vi "Set Z-plane selector disabled state.vi"(8 "error in (no error)":errorcluster, 11 "Functional Imging UI Refs":T1) -> (0 "error out":errorcluster)   [LabVIEW 2013]
uses:
  Typedefs/Functional Imging UI Refs.ctl
  xcontrol/XGrapher.xctl
  Typedefs/ROI selector array-ROI vis.ctl
  xcontrol/Interface VIs/Interface typedefs/Interface-ROI selection cluster.ctl
  Typedefs/ROI ID Enum.ctl
  Typedefs/Groups array referecne.ctl
  Typedefs/ROI visibility mode.ctl
  Global variables/gl_Functional Imaging-Global variables.vi
panel:
  # "[Groups] is a Typedef"
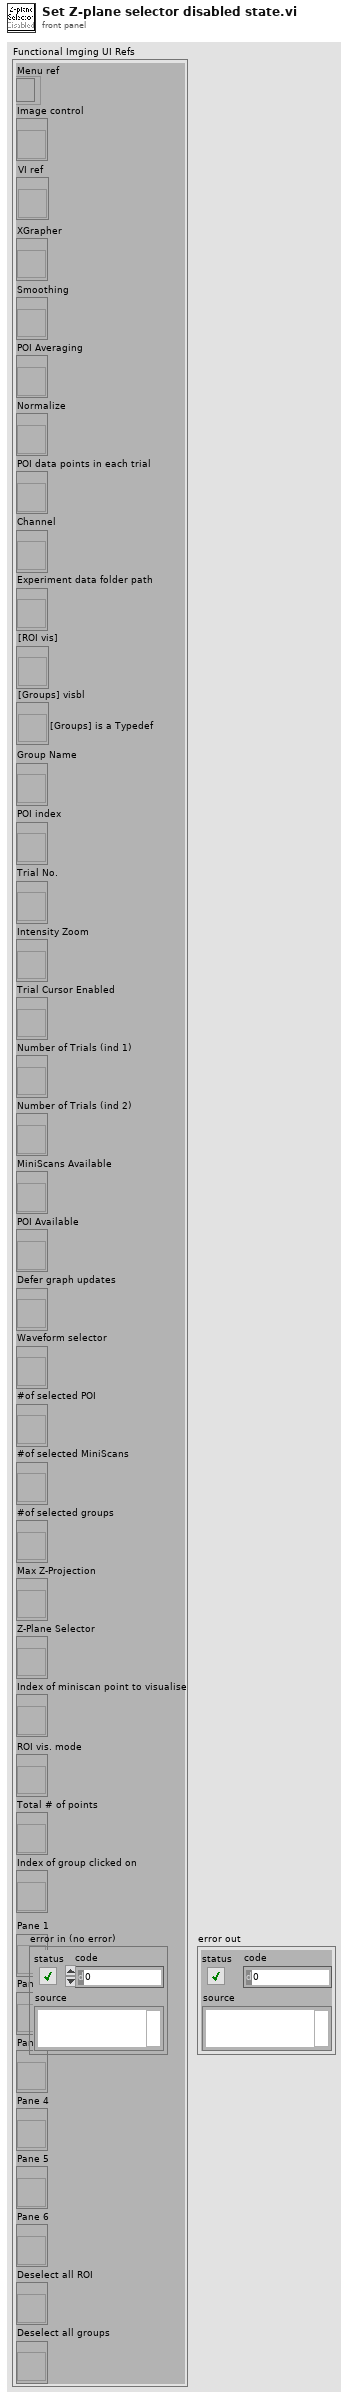
[diagram p1: front panel]
types:
  T1 = typedef "Functional Imging UI Refs.ctl" = cluster{"Menu ref":refnum<k9>, "Image control":refnum<vi>, "VI ref":refnum<vi>, "XGrapher":refnum<vi>, "Smoothing":refnum<vi>, "POI Averaging":refnum<vi>, "Normalize":refnum<vi>, "POI data points in each trial":refnum<vi>, "Channel":refnum<vi>, "Experiment data folder path":refnum<vi>, "[ROI vis]":refnum<vi>, "[Groups] visbl":T2, "Group Name":refnum<vi>, "POI index":refnum<vi>, "Trial No.":refnum<vi>, "Intensity Zoom":refnum<vi>, "Trial Cursor Enabled":refnum<vi>, "Number of Trials (ind 1)":refnum<vi>, "Number of Trials (ind 2)":refnum<vi>, "MiniScans Available":refnum<vi>, "POI Available":refnum<vi>, "Defer graph updates":refnum<vi>, "Waveform selector":refnum<vi>, "#of selected POI":refnum<vi>, "#of selected MiniScans":refnum<vi>, "#of selected groups":refnum<vi>, "Max Z-Projection":refnum<vi>, "Z-Plane Selector":refnum<vi>, "Index of miniscan point to visualise":refnum<vi>, "ROI vis. mode":refnum<vi>, "Total # of points":refnum<vi>, "Index of group clicked on":refnum<vi>, "Pane 1":refnum<vi>, "Pane 2":refnum<vi>, "Pane 3":refnum<vi>, "Pane 4":refnum<vi>, "Pane 5":refnum<vi>, "Pane 6":refnum<vi>, "Deselect all ROI":refnum<vi>, "Deselect all groups":refnum<vi>}
  T2 = typedef "Groups array referecne.ctl" = refnum<vi>
  T3 = enum8{"Enabled", "Disabled", "Disabled and Grayed Out"}
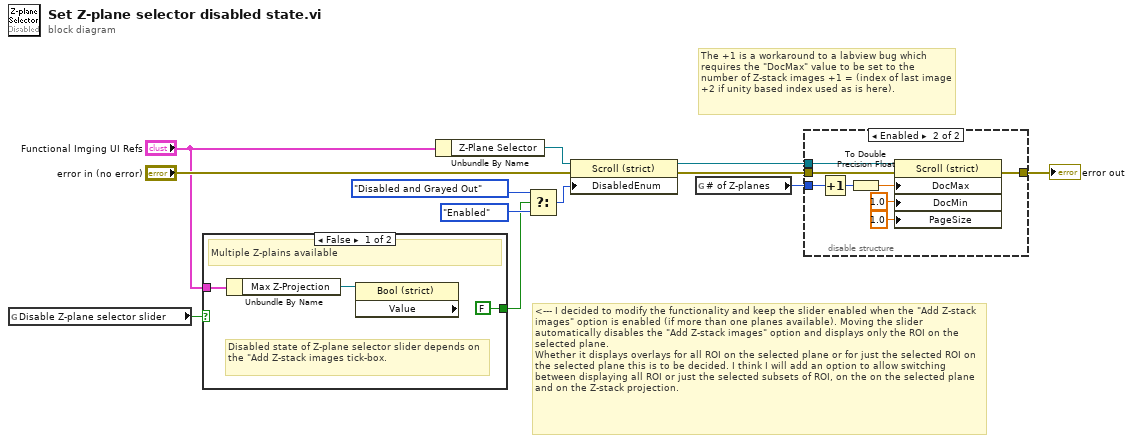
[diagram p0: block diagram]
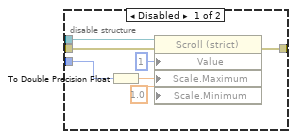
[diagram p2: hidden frame]
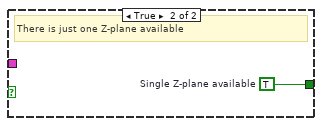
[diagram p3: hidden frame]
diagram:
  # "The +1 is a workaround to a labview bug which requires the \"DocMax\" value to be set to the number of Z-stack images +1 = (index of last image +2 if unity based index used as is here)."
  # "<--- I decided to modify the functionality and keep the slider enabled when the \"Add Z-stack images\" option is enabled (if more than one planes available). Moving the slider automatically disables the \"Add Z-stack images\" option and displays only the ROI on the selected plane.\nWhether it displays overlays for all ROI on the selected plane or for just the selected ROI on the selected plane this is to be decided. I think I will add an option to allow switching between displaying all ROI or just the selected subsets of ROI, on the on the selected plane and on the Z-stack projection."
  n1 = global read "gl_Functional Imaging-Global variables.vi" "Disable Z-plane selector slider"() -> (w6:bool)
  n2 = case shown="False" w6 {
    tunnel: "Functional Imging UI Refs" -> [w14 _]
    tunnel: [FALSE ("Single Z-plane available") w16] -> w5
    frame False {
      # "Disabled state of Z-plane selector slider depends on the \"Add Z-stack images tick-box."
      # "Multiple Z-plains available"
      n3 = Unbundle By Name(w14) -> ("Max Z-Projection"=w15:refnum<vi>)
      n4 = property on="Property Node" class="Bool (strict)" props=["Value"](reference=w15) -> ()  [unwired: 1 in, 3 out]
    }
    frame True {
      w16 = TRUE  # Single Z-plane available
      # "There is just one Z-plane available"
    }
  }
  n5 = Unbundle By Name("Functional Imging UI Refs") -> ("Z-Plane Selector"=w8:refnum<vi>)
  n6 = Select(t=T3."Disabled and Grayed Out" ("Disabled"), s=w5, f=T3."Enabled" ("Disabled")) -> (s? t:f=w11:T3)
  n7 = property on="Property Node" class="Scroll (strict)"(reference=w8, error in="error in (no error)", "DisabledEnum"=w11) -> (reference out=w2:refnum<vi>, error out=w4:errorcluster)
  n8 = global read "gl_Functional Imaging-Global variables.vi" "# of Z-planes"() -> (w1:i32)
  n9 = disable-structure shown="Enabled" {
    disable-tunnel: w4 -> [w23 w31]
    disable-tunnel: [w22 w30] -> w3
    disable-tunnel: w2 -> [w21 w29]
    disable-tunnel: w1 -> [w17 w28]
    frame Disabled {
      n10 = To Double Precision Float(number=w17) -> (double precision float=w18:dbl)
      n11 = property on="Property Node" class="Scroll (strict)"(reference=w21, error in=w23, "Value"=1, "Scale.Maximum"=w18, "Scale.Minimum"=1.0 ("Scale.Range:Minimum")) -> (error out=w22:errorcluster)  [unwired: 1 out]
    }
    frame Enabled {
      n12 = Increment(x=w28) -> (x+1=w25:i32)
      n13 = To Double Precision Float(number=w25) -> (double precision float=w26:dbl)
      n14 = property on="Property Node" class="Scroll (strict)"(reference=w29, error in=w31, "DocMax"=w26, "DocMin"=1.0 ("Scale.Range:Minimum"), "PageSize"=1.0 ("Page Size")) -> (error out=w30:errorcluster)  [unwired: 1 out]
    }
  }
  "error out" <- w3
